vi "Clamp AET Min_Horizontal.vi"(0 "Image":T4, 1 "Rectangle":T8 {"Rotation" format="%.2f"; "Left" scale=0.0..1024.0; "Right" scale=0.0..1024.0}, 4 "Coordinate System":T7 {"Measurement System"."Axis Reference" items=["Direct", "Indirect"]; "Measurement System"."Angle (deg)" format="%.2f"; "Measurement System"."Origin"."Y" format="%.2f"; "Measurement System"."Origin"."X" format="%.2f"; "Reference System"."Axis Reference" items=["Direct", "Indirect"]; "Reference System"."Angle (deg)" format="%.2f"; "Reference System"."Origin"."Y" format="%.2f"; "Reference System"."Origin"."X" format="%.2f"}, 5 "error in (no error)":errorcluster, 6 "Settings":T3={"Contrast"=40, "Filter width"=4, "Steepness"=2, "Subsampling Ratio"=5, "Show Search Area"=FALSE, "Show Search Lines"=FALSE, "Show Edges Found"=FALSE, "Show Result"=TRUE}, 7 "Edge Options":T5={"Edge Polarity"=0, "Kernel Size"=3, "Width"=3, "Minimum Edge Strength"=10.0, "Interpolation Type"=enum."Bilinear Fixed", "Data Processing Method"=enum."Average"} {"Edge Polarity" items=["All Edges", "Rising Edges", "Falling Edges"]; "Minimum Edge Strength" format="%.2f"; "Width" step=2; "Kernel Size" step=2}) -> (11 "First Edges 2":T1[](array[typedef]) {"Distance (Real-World)" format="%.2f"; "Location (Real-World)"."Y" format="%.2g"; "Location (Real-World)"."X" format="%.2f"; "Noise" format="%.2f"; "Location (Pixel)"."Y" format="%.2g"; "Location (Pixel)"."X" format="%.2f"; "Strength" format="%.2f"; "Distance (Pixel)" format="%.2f"}, 12 "Edge Coordinates":cluster{"X":sgl, "Y":sgl}[](array[cluster]) {"Y" format="%.2f"; "X" format="%.2f"}, 13 "Search Lines":T2[](array[typedef]) {"Edge Info"."Distance (Real-World)" format="%.2f"; "Edge Info"."Location (Real-World)"."Y" format="%.2g"; "Edge Info"."Location (Real-World)"."X" format="%.2f"; "Edge Info"."Noise" format="%.2f"; "Edge Info"."Location (Pixel)"."Y" format="%.2g"; "Edge Info"."Location (Pixel)"."X" format="%.2f"; "Edge Info"."Strength" format="%.2f"; "Edge Info"."Distance (Pixel)" format="%.2f"}, 14 "Image Out":T4, 15 "Distance":sgl format="%.2f", 16 "First Edges":T1[](array[typedef]) {"Distance (Real-World)" format="%.2f"; "Location (Real-World)"."Y" format="%.2g"; "Location (Real-World)"."X" format="%.2f"; "Noise" format="%.2f"; "Location (Pixel)"."Y" format="%.2g"; "Location (Pixel)"."X" format="%.2f"; "Strength" format="%.2f"; "Distance (Pixel)" format="%.2f"}, 17 "First and Last Edge Points":cluster{"X":sgl, "Y":sgl}[](array[cluster]), 18 "Coordinate System (duplicate)":T7 {"Measurement System"."Axis Reference" items=["Direct", "Indirect"]; "Measurement System"."Angle (deg)" format="%.2f"; "Measurement System"."Origin"."Y" format="%.2f"; "Measurement System"."Origin"."X" format="%.2f"; "Reference System"."Axis Reference" items=["Direct", "Indirect"]; "Reference System"."Angle (deg)" format="%.2f"; "Reference System"."Origin"."Y" format="%.2f"; "Reference System"."Origin"."X" format="%.2f"}, 19 "error out":errorcluster)   [LabVIEW 2019, in "Algorithm.lvclass"]
doc: "Modified NI Horizontal Min Clamp with Rake-3 which uses Advanced Edge Detection"
uses:
  FrameworkOverrides/Algorithm.lvclass
  <vilib>/vision/NI_Vision_Development_Module.lvlib
  <vilib>/vision/Image Controls.llb/IMAQ Image.ctl
  <vilib>/vision/Measure.llb/Edge Polarity.ctl
  <vilib>/vision/Measure.llb/Edge Options.ctl
  <vilib>/vision/Measure.llb/Edge New.ctl
  <vilib>/vision/Measure.llb/Search Line.ctl
panel:
  out "Elapsed time (ms)":u32
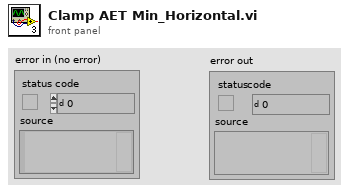
[diagram p1: front panel]
types:
  T1 = typedef "Edge New.ctl" = cluster{"Location (Pixel)":cluster{"X":sgl, "Y":sgl}, "Location (Real-World)":cluster{"X":sgl, "Y":sgl}, "Distance (Pixel)":dbl, "Distance (Real-World)":dbl, "Strength":dbl, "Noise":dbl, "Rising?":bool}
  T2 = typedef "Search Line.ctl" = cluster{"Start Point":cluster{"X":sgl, "Y":sgl}, "End Point":cluster{"X":sgl, "Y":sgl}, "Edge Info":T1[], "Edge Map":dbl[], "Calibration Valid":bool}
  T3 = cluster{"Contrast":i32, "Filter width":i32, "Steepness":i32, "Subsampling Ratio":u32, "Show Search Area":bool, "Show Search Lines":bool, "Show Edges Found":bool, "Show Result":bool}
  T4 = typedef "IMAQ Image.ctl" = refnum<image>
  T5 = typedef "Edge Options.ctl" = cluster{"Edge Polarity":T6, "Kernel Size":u32, "Width":u32, "Minimum Edge Strength":sgl, "Interpolation Type":enum32{"Zero Order", "Bilinear", "Quadratic", "Cubic", "Bilinear Fixed"}, "Data Processing Method":enum32{"Average", "Median"}}
  T6 = typedef "Edge Polarity.ctl" = u32
  T7 = typedef "IMAQ Coordinate System" = cluster{"Reference System":cluster{"Origin":cluster{"X":sgl, "Y":sgl}, "Angle (deg)":sgl, "Axis Reference":u32}, "Measurement System":cluster{"Origin":cluster{"X":sgl, "Y":sgl}, "Angle (deg)":sgl, "Axis Reference":u32}}
  T8 = typedef "IMAQ Rectangle" = cluster{"Left":i32, "Top":i32, "Right":i32, "Bottom":i32, "Rotation":dbl}
  T9 = cluster{"Start Point":cluster{"X":sgl, "Y":sgl}, "End Point":cluster{"X":sgl, "Y":sgl}}
  T10 = typedef "ROI Descriptor" = cluster{"Global Rectangle":i32[], "Contours":cluster{"ID":enum32{"External", "Internal"}, "Type":u32, "Coordinates":i32[]}[]}
  T11 = cluster{"Global Rectangle":i32[], "Contours":cluster{"ID":enum32{"External", "Internal"}, "Type":u32, "Coordinates":i32[]}[]}
  T12 = enum32{"Get First Edge", "Get First + Last Edge", "Get All Edges"}
  T13 = cluster{"End Point":cluster{"X":sgl, "Y":sgl}, "End Point":cluster{"X":sgl, "Y":sgl}}
  T14 = cluster{cluster{"X":sgl, "Y":sgl}, cluster{"X":sgl, "Y":sgl}}[]
  T15 = cluster{"Show Search Area":bool, "Show Search Lines":bool, "Show Edges Found":bool, "Show Result":bool}
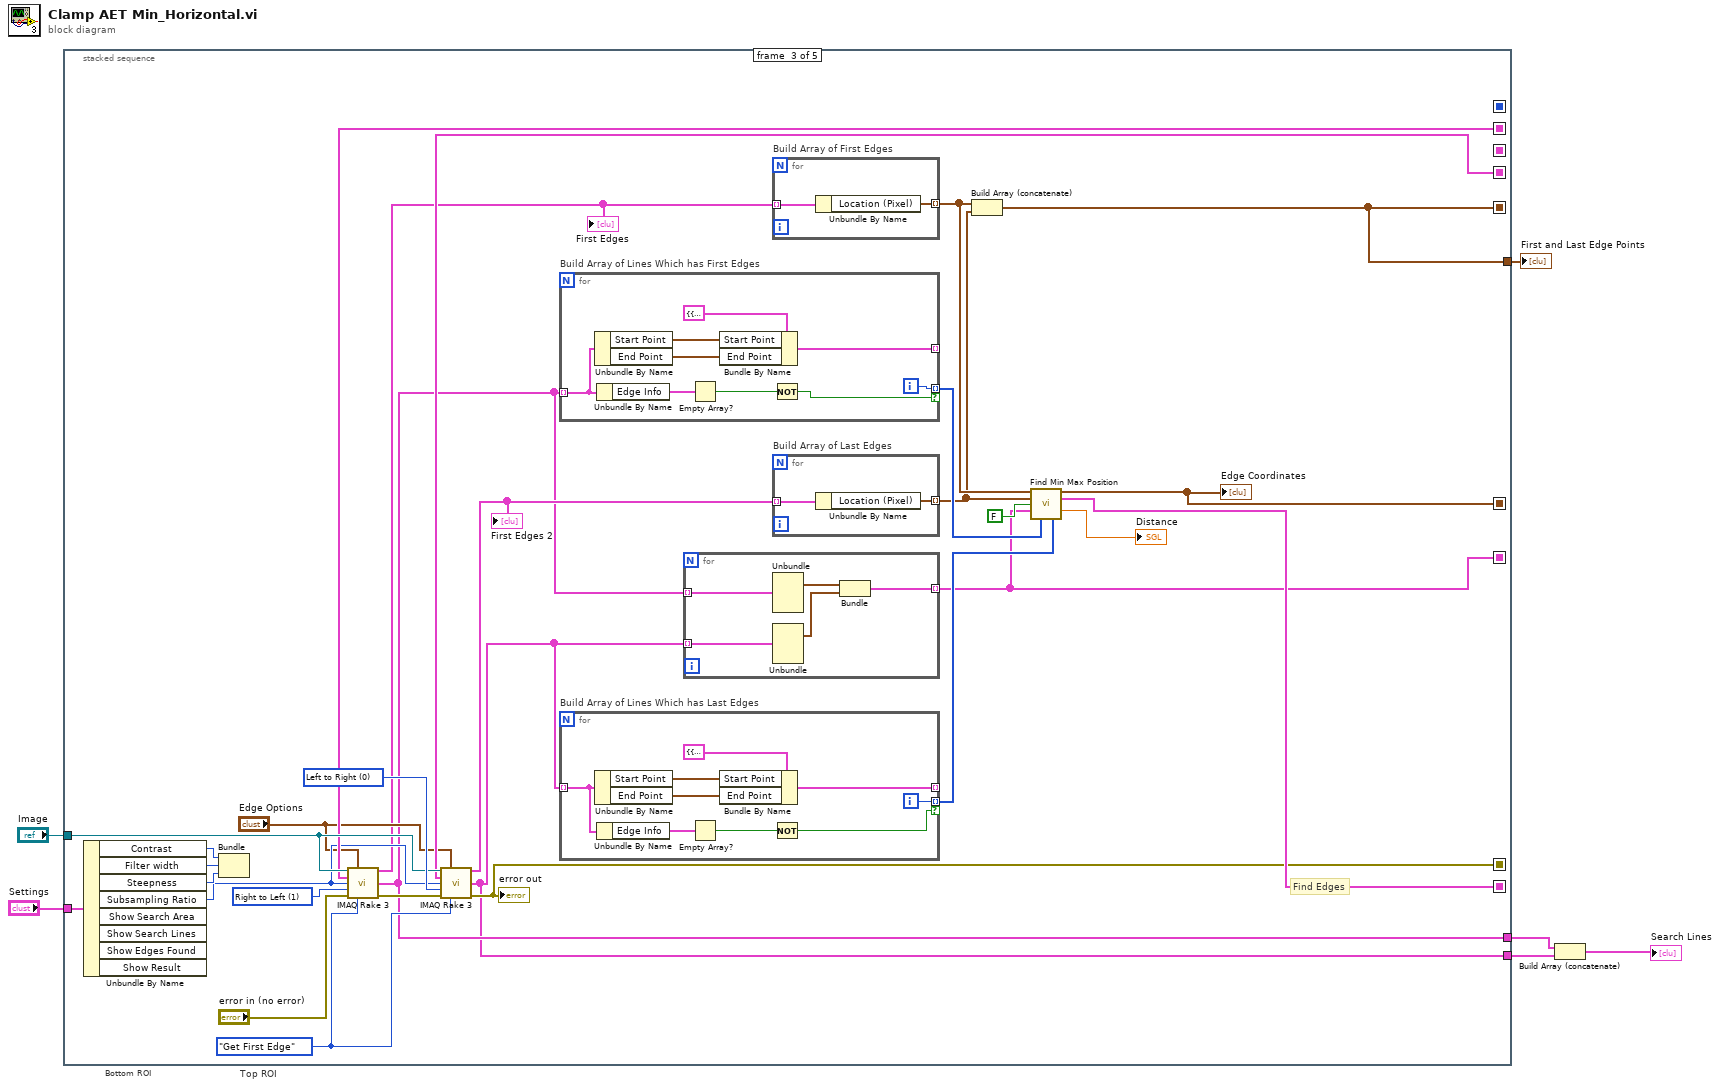
[diagram p0: block diagram]
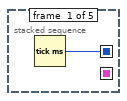
[diagram p2: hidden frame]
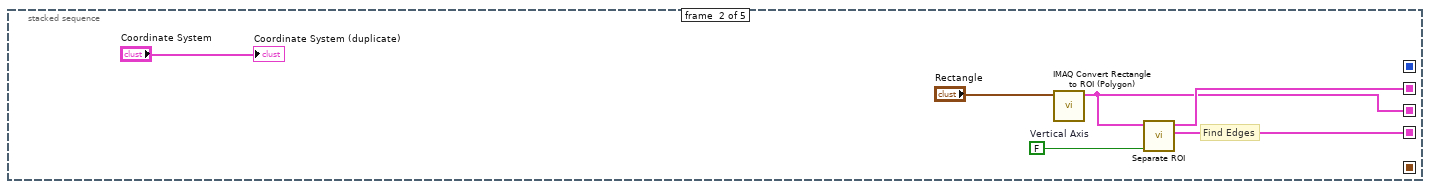
[diagram p3: hidden frame]
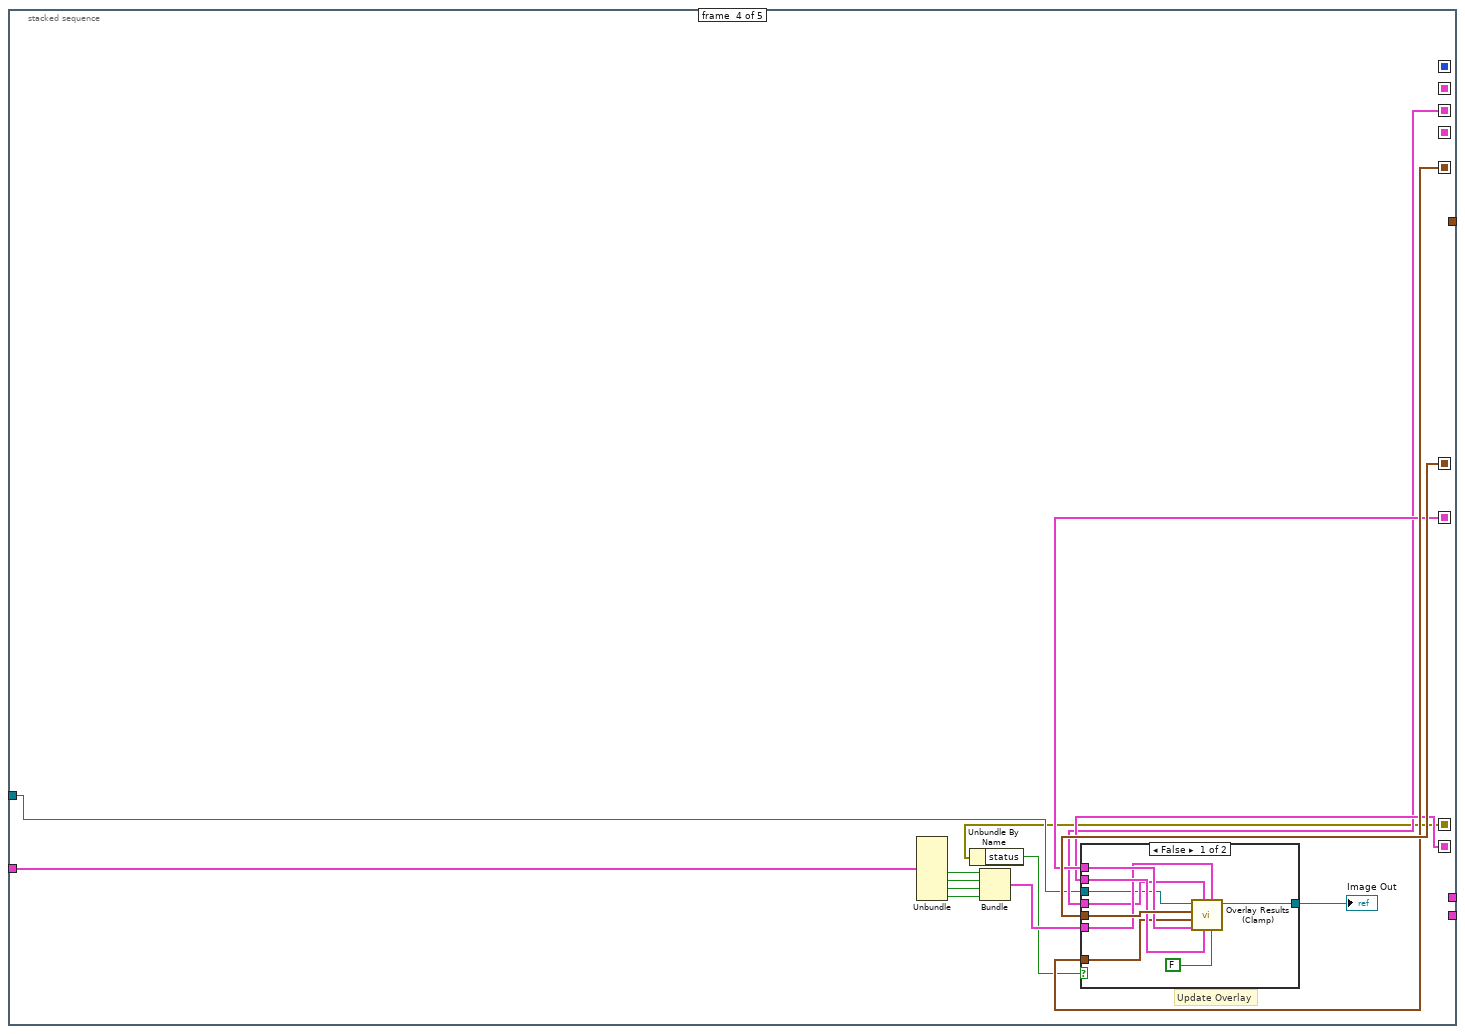
[diagram p4: hidden frame]
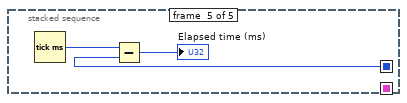
[diagram p6: hidden frame]
diagram:
  # "Bottom ROI"
  # "Top ROI"
  n1 = stacked-sequence {
    seq-local: [_ _ w36 _ _] -> [_ _ _ w84 _]
    seq-local: [w7 _ _ _ _] -> [_ _ _ _ w97]
    seq-local: [_ _ w16 _ _] -> [_ _ _ w83 _]
    seq-local: [_ _ w17 _ _] -> [_ _ _ w82 _]
    seq-local: [_ _ w37 _ _] -> [_ _ _ w76 _]
    seq-local: [_ w12 _ _ _] -> [_ _ w28 _ _]
    seq-local: [_ w11 _ _ _] -> [_ _ w27 _ _]
    seq-local: [_ w8 _ _ _] -> [_ _ _ w74 _]
    seq-local: [_ _ w25 _ _] -> [_ _ _ w71 _]
    tunnel: "Image" -> [_ _ w31 w73 _]
    tunnel: "Settings" -> [_ _ w38 w77 _]
    tunnel: [_ _ w16 _ _] -> w4
    tunnel: [_ _ w15 _ _] -> w3
    tunnel: [_ _ w14 _ _] -> w2
    frame #0 {
      n2 = Tick Count (ms)() -> (millisecond timer value=w7:u32)
    }
    frame #1 {
      w10 = FALSE  # Vertical Axis
      # "Find Edges"
      n3 = call "IMAQ Convert Rectangle to ROI (Polygon)"("Rectangle"="Rectangle") -> ("ROI Descriptor"=w8:T10)  [unwired: 1 in, 8 out]
      n4 = call <vilib>:"Separate ROI.vi"("Axis"=w10, "ROI Descriptor"=w8) -> ("Right/Bottom ROI"=w11:T11, "Left/Top ROI"=w12:T11)  [unwired: 4 out]
      "Coordinate System (duplicate)" <- "Coordinate System"
    }
    frame #2 {
      w32 = u32 0 items=["Left to Right", "Right to Left", "Top to Bottom", "Bottom to Top"]
      w34 = T12."Get First Edge" ("Process")
      w33 = u32 1 items=["Left to Right", "Right to Left", "Top to Bottom", "Bottom to Top"]
      # "Find Edges"
      n5 = Unbundle By Name(w38) -> ("Contrast"=w40:i32, "Filter width"=w41:i32, "Steepness"=w42:i32, "Subsampling Ratio"=w26:u32)  [unwired: 4 out]
      n6 = Bundle("Contrast"=w40, "Filter width"=w41, "Steepness"=w42) -> ()  [unwired: 2 out]
      n7 = call "IMAQ Rake 3"("Image"=w31, "Edge Options"="Edge Options", "ROI Descriptor"=w28, "Step Size"=w26, "Scan Direction"=w33, "error in (no error)"="error in (no error)", "Process"=w34) -> ("First Edges"=w21:T1[], "Search Lines"=w15:T2[], "error out"=w29:errorcluster)  [unwired: 5 in, 1 out]
      "First Edges" <- w21
      n8 = call "IMAQ Rake 3"("Image"=w31, "Edge Options"="Edge Options", "ROI Descriptor"=w27, "Step Size"=w26, "Scan Direction"=w32, "error in (no error)"=w29, "Process"=w34) -> ("First Edges"=w20:T1[], "Search Lines"=w14:T2[], "error out"=w25:errorcluster)  [unwired: 5 in, 1 out]
      "error out" <- w25
      "First Edges 2" <- w20
      n9 = for "Build Array of Lines Which has First Edges" {
        tunnel: w15 -> [w61] mode=indexing
        tunnel: [w62] -> _ mode=indexing
        tunnel: [w58] -> w24 mode=indexing if=w57
        i -> [w58]
        n10 = Unbundle By Name(w61) -> ("Start Point"=w64:cluster{"X":sgl, "Y":sgl}, "End Point"=w63:cluster{"X":sgl, "Y":sgl})
        n11 = Unbundle By Name(w61) -> ("Edge Info"=w60:T1[])
        n12 = Empty Array?(array=w60) -> (empty?=w59:bool)
        n13 = Bundle By Name(cluster=T9 {"Start Point"={"X"=0.0, "Y"=0.0}, "End Point"={"X"=0.0, "Y"=0.0}} ("Cluster 2"), "Start Point"=w64, "End Point"=w63) -> (w62:T9)
        n14 = Not(x=w59) -> (.not. x?=w57:bool)
      }
      n15 = for "Build Array of Lines Which has Last Edges" {
        tunnel: [w53] -> _ mode=indexing
        tunnel: [w50] -> w23 mode=indexing if=w49
        tunnel: w14 -> [w47] mode=indexing
        i -> [w50]
        n16 = Unbundle By Name(w47) -> ("Start Point"=w55:cluster{"X":sgl, "Y":sgl}, "End Point"=w54:cluster{"X":sgl, "Y":sgl})
        n17 = Unbundle By Name(w47) -> ("Edge Info"=w52:T1[])
        n18 = Empty Array?(array=w52) -> (empty?=w51:bool)
        n19 = Bundle By Name(cluster=T9 {"Start Point"={"X"=0.0, "Y"=0.0}, "End Point"={"X"=0.0, "Y"=0.0}} ("Cluster 2"), "Start Point"=w55, "End Point"=w54) -> (w53:T9)
        n20 = Not(x=w51) -> (.not. x?=w49:bool)
      }
      n21 = for {
        tunnel: w15 -> [w69] mode=indexing
        tunnel: w14 -> [w68] mode=indexing
        tunnel: [w65] -> w17 mode=indexing
        n22 = Unbundle(w69) -> ("End Point"=w67:cluster{"X":sgl, "Y":sgl})  [unwired: 4 out]
        n23 = Unbundle(w68) -> ("End Point"=w66:cluster{"X":sgl, "Y":sgl})  [unwired: 4 out]
        n24 = Bundle("End Point"=w67, "End Point"=w66) -> (w65:T13)  [unwired: 1 out]
      }
      n25 = for "Build Array of First Edges" {
        tunnel: w21 -> [w46] mode=indexing
        tunnel: [w45] -> w19 mode=indexing
        n26 = Unbundle By Name(w46) -> ("Location (Pixel)"=w45:cluster{"X":sgl, "Y":sgl})
      }
      n27 = for "Build Array of Last Edges" {
        tunnel: w20 -> [w44] mode=indexing
        tunnel: [w43] -> w18 mode=indexing
        n28 = Unbundle By Name(w44) -> ("Location (Pixel)"=w43:cluster{"X":sgl, "Y":sgl})
      }
      n29 = Build Array (concatenate)(w19, w18) -> (w16:cluster{"X":sgl, "Y":sgl}[])
      n30 = call "Find Min Max Position.vi"("First Edges"=w19, "Last Edges"=w18, "Min / Max"=FALSE, "Search Lines"=w17, "Lines with Edges (first)"=w24, "Lines with Edges (last)"=w23) -> ("Points"=w36:cluster{"X":sgl, "Y":sgl}[], "Perpendicular Lines"=w37:T14, "Distance"=→"Distance":sgl)  [unwired: 6 in, 1 out]
      "Edge Coordinates" <- w36
    }
    frame #3 {
      # "Update Overlay"
      n31 = Unbundle(w77) -> ("Show Search Area"=w81:bool, "Show Search Lines"=w80:bool, "Show Edges Found"=w79:bool, "Show Result"=w78:bool)  [unwired: 4 out]
      n32 = Unbundle By Name(w71) -> ("status"=w70:bool)
      n33 = Bundle("Show Search Area"=w81, "Show Search Lines"=w80, "Show Edges Found"=w79, "Show Result"=w78) -> (w75:T15)  [unwired: 1 out]
      n34 = case shown="False" w70 {
        tunnel: w84 -> [w93 _]
        tunnel: w83 -> [w85 _]
        tunnel: w82 -> [w92 _]
        tunnel: w76 -> [w91 _]
        tunnel: w75 -> [w89 _]
        tunnel: w74 -> [w88 _]
        tunnel: w73 -> [w87 w94]
        tunnel: [w86 w94] -> w72
        frame False {
          n35 = call <vilib>:"Overlay Results (Clamp).vi"("Min / Max"=FALSE, "Setup"=w89, "Perpendicular Lines"=w91, "ROI Descriptor"=w88, "Search Lines"=w92, "All Edges Found"=w85, "Measurement Edges"=w93, "Image In"=w87) -> ("Image Out"=w86:T4)  [unwired: 3 out]
        }
        frame True {
        }
      }
      "Image Out" <- w72
    }
    frame #4 {
      n36 = Tick Count (ms)() -> (millisecond timer value=w96:u32)
      n37 = Subtract(x=w96, y=w97) -> (x-y=→"Elapsed time (ms)":u32)
    }
  }
  "First and Last Edge Points" <- w4
  n38 = Build Array (concatenate)(w3, w2) -> (→"Search Lines":T2[])
